vi "HOST - DRAM FIFO test with data.vi"() -> ()   [LabVIEW 2019]
uses:
  <vilib>/rvi/interface/nirviOpenFPGA/nirviOpenFPGA.xnode
  FPGA Bitfiles/DRAM_FIFO_test_with_data_v2.lvbitx
  <vilib>/rvi/interface/nirviReadWriteControl/nirviReadWriteControl.xnode
  NiFpgaLv.dll
  <vilib>/Utility/error.llb/Error Cluster From Error Code.vi
  <vilib>/rvi/interface/Simulation/niFpgaSimulationCallBeginRW.vi
  <vilib>/rvi/errors/niLvFpgaAdjustHostInterfaceError.vi
  e19cebdc-8c77-453c-97e0-e94ec5b4f09b.vi
  <vilib>/rvi/interface/nirviMethod/nirviMethod.xnode
  <vilib>/FPGAPlugInAG/Dynamic/niLvFpga_ConfigureFifo_Dynamic.vi
  <vilib>/rvi/errors/niLvFpgaMergeErrorWithErrorCode.vi
  <vilib>/rvi/interface/nirviCloseFPGA/nirviCloseFPGA.xnode
  <vilib>/FPGAPlugInAG/Dynamic/niLvFpga_ReadFifo_Dynamic.vi
  <vilib>/Analysis/NI_AALBase.lvlib
  <vilib>/FPGAPlugInAG/PXIe-7902R/niLvFpga_Open_PXIe-7902R.vi
  <vilib>/rvi/interface/common/dynamic/niFpgaDynamicAddResources.vi
  <vilib>/FPGAPlugInAG/Dynamic/niLvFpga_WriteFifo_Dynamic.vi
  <vilib>/FPGAPlugInAG/Dynamic/niLvFpga_Close_Dynamic.vi
  <vilib>/userdefined/High Color/nirio_resource_hc.ctl
panel:
  out "status 2":T1
  out "Array":fxp<+/-,12,1>[](array[numeric])
  out "initialized array":fxp<+/-,12,1>[](array[numeric])
  out "Empty Elements Remaining":u32
  in  "start acq":bool
  in  "size":i32 format="%#_3p"
  out "status":string
  out "DRAM overflow":bool
  out "DRAM highwater":u32
  out "samples available":u32
  in  "retrieve":bool
  in  "download data":bool
  in  "stop":bool
  in  "resource name":T2
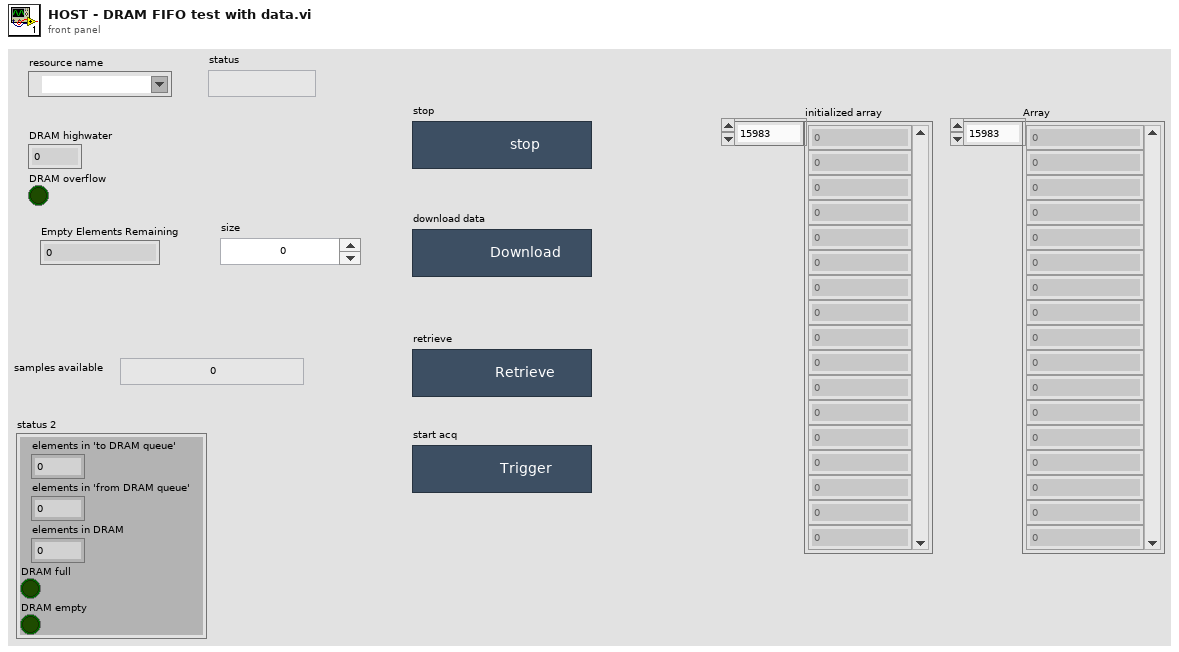
[diagram p1: front panel]
types:
  T1 = cluster{"elements in 'to DRAM queue'":u32, "elements in 'from DRAM queue'":u32, "elements in DRAM":u32, "DRAM full":bool, "DRAM empty":bool}
  T2 = typedef "nirio_resource_hc.ctl" = tag
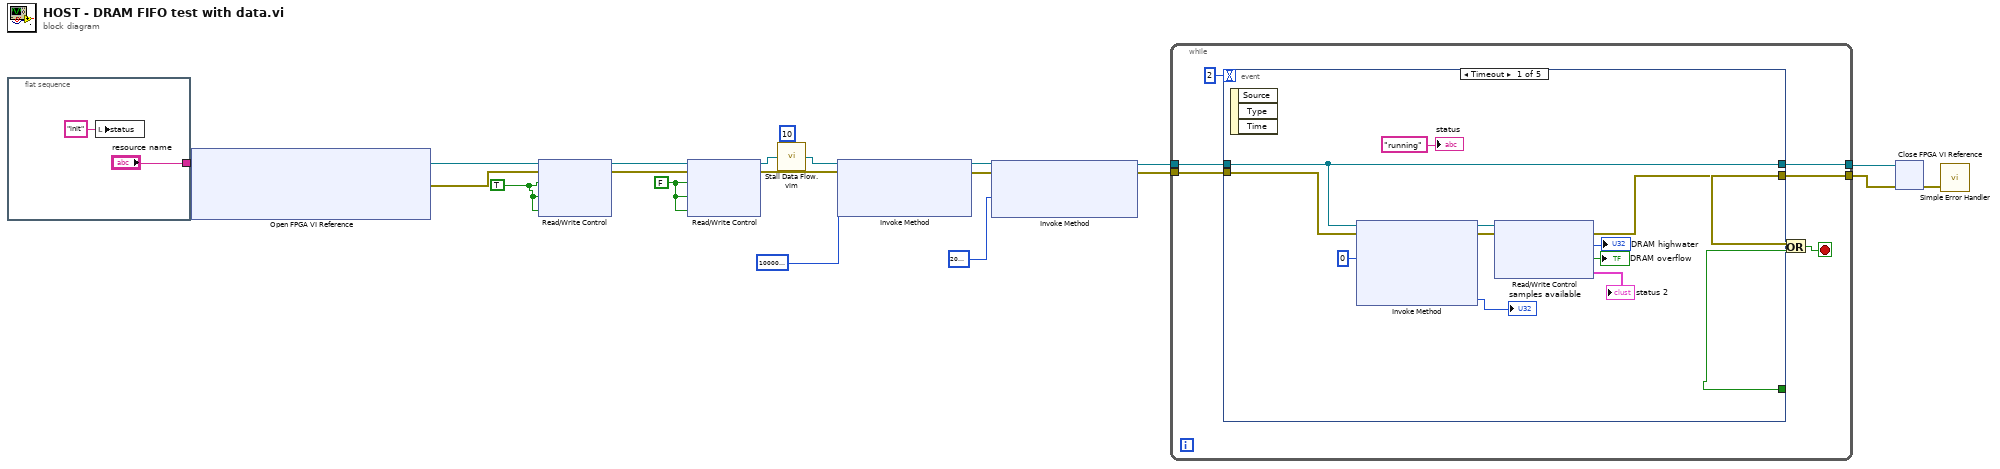
[diagram p0: block diagram]
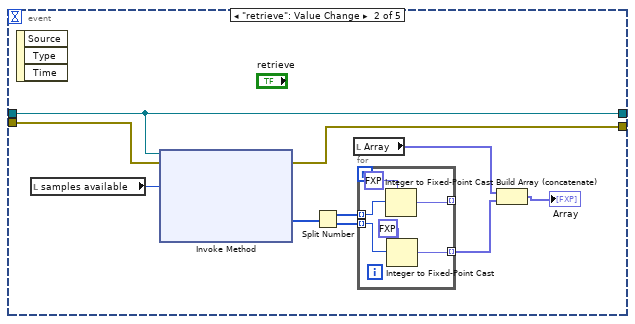
[diagram p2: hidden frame]
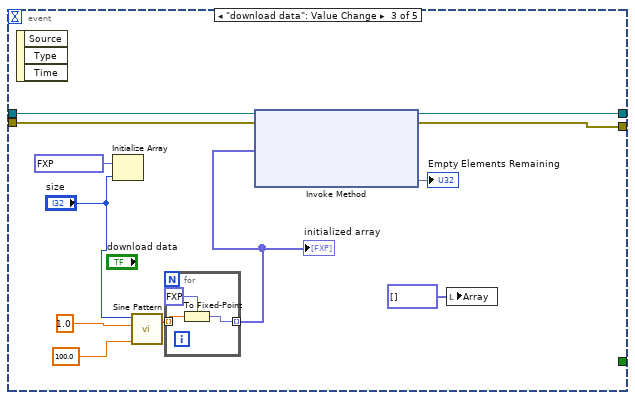
[diagram p3: hidden frame]
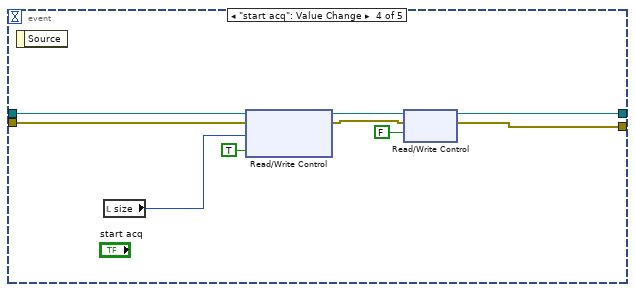
[diagram p4: hidden frame]
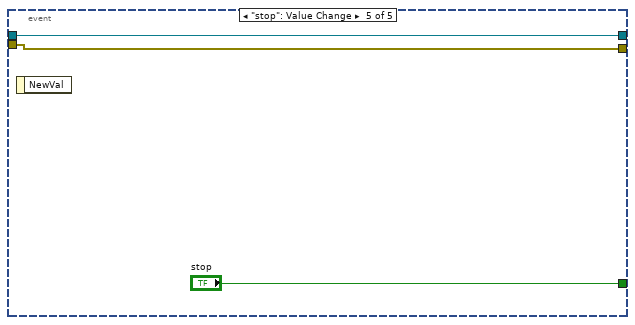
[diagram p5: hidden frame]
diagram:
  w14 = FALSE
  w18 = TRUE ("reset")
  n1 = flat-sequence {
    tunnel: ["resource name"] -> w20
    frame #0 {
      n2 = local write "status"("init" ("status")) -> ()
    }
  }
  n3 = xnode "Open FPGA VI Reference"("resource name"=w20) -> ("FPGA VI Reference Out"=w19:refnum<k20>, "error out"=w17:errorcluster)  [unwired: 1 in]
  n4 = xnode "Read/Write Control"("FPGA VI Reference In"=w19, "error in"=w17, "reset"=w18, "reset DRAM"=w18, "dram.flush"=w18) -> ("FPGA VI Reference Out"=w16:refnum<k20>, "error out"=w15:errorcluster)
  n5 = xnode "Read/Write Control"("FPGA VI Reference In"=w16, "error in"=w15, "reset"=w14, "reset DRAM"=w14, "dram.flush"=w14) -> ("FPGA VI Reference Out"=w13:refnum<k20>, "error out"=w11:errorcluster)
  n6 = call "Stall Data Flow.vim"("value in"=w13, "milliseconds to wait"=u32 10) -> ("value out"=w10:refnum<k20>)  [unwired: 1 out]
  n7 = xnode "Invoke Method"("FPGA VI Reference In"=w10, "error in"=w11, "Requested Depth"=u32 100000000) -> ("FPGA VI Reference Out"=w9:refnum<k20>, "error out"=w8:errorcluster)  [unwired: 1 out]
  n8 = xnode "Invoke Method"("FPGA VI Reference In"=w9, "error in"=w8, "Requested Depth"=u32 2000000) -> ("FPGA VI Reference Out"=w6:refnum<k20>, "error out"=w5:errorcluster)  [unwired: 1 out]
  n9 = while {
    tunnel: w6 -> [w28]
    tunnel: w5 -> [w27]
    tunnel: [w26] -> w4
    tunnel: [w25] -> w3
    stop <- w23 stop-if-true
    n10 = event shown="[0] Timeout" {
      selector: _ -> [_ _ _ _ _]
      dyn-events: _ -> [_ _ _ _ _]
      timeout: 2 -> [_ _ _ _ _]
      tunnel: [_ _ _ _ "stop"] -> w24
      tunnel: w28 -> [w31 w50 w68 w80 w82]
      tunnel: w27 -> [w40 w48 w66 w75 w81]
      tunnel: [w31 w50 w67 w76 w82] -> w26
      tunnel: [w35 w47 w65 w73 w81] -> w25
      event Timeout {
        n11 = event-data() -> ()  [unwired: 1 in, 3 out]
        n12 = xnode "Invoke Method"("FPGA VI Reference In"=w31, "error in"=w40, "Number of Elements"=u32 0) -> ("FPGA VI Reference Out"=w36:refnum<k20>, "error out"=w37:errorcluster, "Elements Remaining"=→"samples available":u32)  [unwired: 1 in, 1 out]
        n13 = xnode "Read/Write Control"("FPGA VI Reference In"=w36, "error in"=w37) -> ("error out"=w35:errorcluster, "DRAM highwater"=→"DRAM highwater":u32, "DRAM overflow"=→"DRAM overflow":bool, "status"=→"status 2":T1)  [unwired: 1 out]
        "status" <- "running" ("status")
      }
      event "retrieve": Value Change {
        n14 = event-data() -> ()  [unwired: 1 in, 3 out]
        n15 = local read "samples available"() -> (w49:u32)
        n16 = xnode "Invoke Method"("FPGA VI Reference In"=w50, "error in"=w48, "Number of Elements"=w49) -> ("error out"=w47:errorcluster, "Data"=w46:u32[])  [unwired: 1 in, 2 out]
        n17 = Split Number(x=w46) -> (hi(x)=w45:u16[], lo(x)=w44:u16[])
        n18 = local read "Array"() -> (w42:fxp<+/-,12,1>[])
        n19 = for {
          tunnel: w45 -> [w56] mode=indexing
          tunnel: w44 -> [w55] mode=indexing
          tunnel: [w52] -> _ mode=indexing
          tunnel: [w51] -> w41 mode=indexing
          n20 = Integer to Fixed-Point Cast(fixed-point type=fxp<+/-,12,1> 0.0 ("element"), integer=w56) -> (fixed-point=w52:fxp<+/-,12,1>)
          n21 = Integer to Fixed-Point Cast(fixed-point type=fxp<+/-,12,1> 0.0 ("element"), integer=w55) -> (fixed-point=w51:fxp<+/-,12,1>)
        }
        n22 = Build Array (concatenate)(w42, w41) -> (→"Array":fxp<+/-,12,1>[])
      }
      event "download data": Value Change {
        n23 = event-data() -> ()  [unwired: 1 in, 3 out]
        n24 = Initialize Array(fxp<+/-,12,1> 0.009765625 ("element"), "size") -> ()  [unwired: 1 out]
        n25 = call <vilib>:"Sine Pattern.vi"("cycles"=100.0, "amplitude"=1.0, "samples"="size") -> ("Sinusoidal Pattern"=w58:dbl[])  [unwired: 1 in, 1 out]
        n26 = for {
          tunnel: w58 -> [w71] mode=indexing
          tunnel: [w69] -> w57 mode=indexing
          n27 = To Fixed-Point(fixed-point type=fxp<+/-,12,1> 0.0 ("element"), number=w71) -> (fixed-point=w69:fxp<+/-,12,1>)
        }
        "initialized array" <- w57
        n28 = xnode "Invoke Method"("FPGA VI Reference In"=w68, "error in"=w66, "Data"=w57) -> ("FPGA VI Reference Out"=w67:refnum<k20>, "error out"=w65:errorcluster, "Empty Elements Remaining"=→"Empty Elements Remaining")  [unwired: 1 in]
        n29 = local write "Array"(fxp<+/-,12,1>[] [] ("Array")) -> ()
      }
      event "start acq": Value Change {
        n30 = event-data() -> ()  [unwired: 1 in, 1 out]
        n31 = local read "size"() -> (w72:i32)
        n32 = xnode "Read/Write Control"("FPGA VI Reference In"=w80, "error in"=w75, "signal length"=w72, "start"=TRUE) -> ("FPGA VI Reference Out"=w78:refnum<k20>, "error out"=w74:errorcluster)
        n33 = xnode "Read/Write Control"("FPGA VI Reference In"=w78, "error in"=w74, "start"=FALSE) -> ("FPGA VI Reference Out"=w76:refnum<k20>, "error out"=w73:errorcluster)
      }
      event "stop": Value Change {
        n34 = event-data() -> ()  [unwired: 1 in, 1 out]
      }
    }
    n35 = Or(x=w25, y=w24) -> (x .or. y?=w23:bool)
  }
  n36 = xnode "Close FPGA VI Reference"("FPGA VI Reference In"=w4, "error in"=w3) -> ("error out"=w2:errorcluster)
  n37 = call <vilib>:"Simple Error Handler.vi"("error in (no error)"=w2) -> ()  [unwired: 4 in, 5 out]
